vi "PenaltyAttackerRole.vi"(8 "error in (no error)":errorcluster, 9 "Robot in":refnum<class "Robot.lvclass">, 10 "Game in":refnum<class "Game.lvclass">, 11 "PenaltyAttackerRole in":refnum<class "PenaltyAttackerRole.lvclass">) -> (0 "error out":errorcluster, 2 "Robot out":refnum<class "Robot.lvclass">, 3 "PenaltyAttackerRole out":refnum<class "PenaltyAttackerRole.lvclass">)   [LabVIEW 2018, in "PenaltyAttackerRole.lvclass"]
uses:
  PenaltyAttackerRole.lvclass
  C:/Users/Gustavo/Desktop/RoboIMEINTEL/SSL_AI/Role_class/Role.lvclass
  Robot_class/Robot.lvclass
  Game_class/Game.lvclass
  Role_class/Role.lvclass/Role.ctl
  Tacticbook_class/Tacticbook.lvclass/Tacticbook.ctl
  Tacticbook_class/Read PenaltyAttackerTactic.vi
  PenaltyAttackerTactic_class/Read States.vi
  Tacticbook_class/Write PenaltyAttackerTactic.vi
  Role_class/Read Tacticbook.vi
  Role_class/Read tactic_index.vi
  Role_class/Write Tacticbook.vi
  Role_class/Write tactic_index.vi
  Tacticbook_class/Tacticbook.lvclass
  PenaltyAttackerTactic_class/PenaltyAttackerTactic.lvclass
panel:
  out "Game out":refnum<class "Game.lvclass">
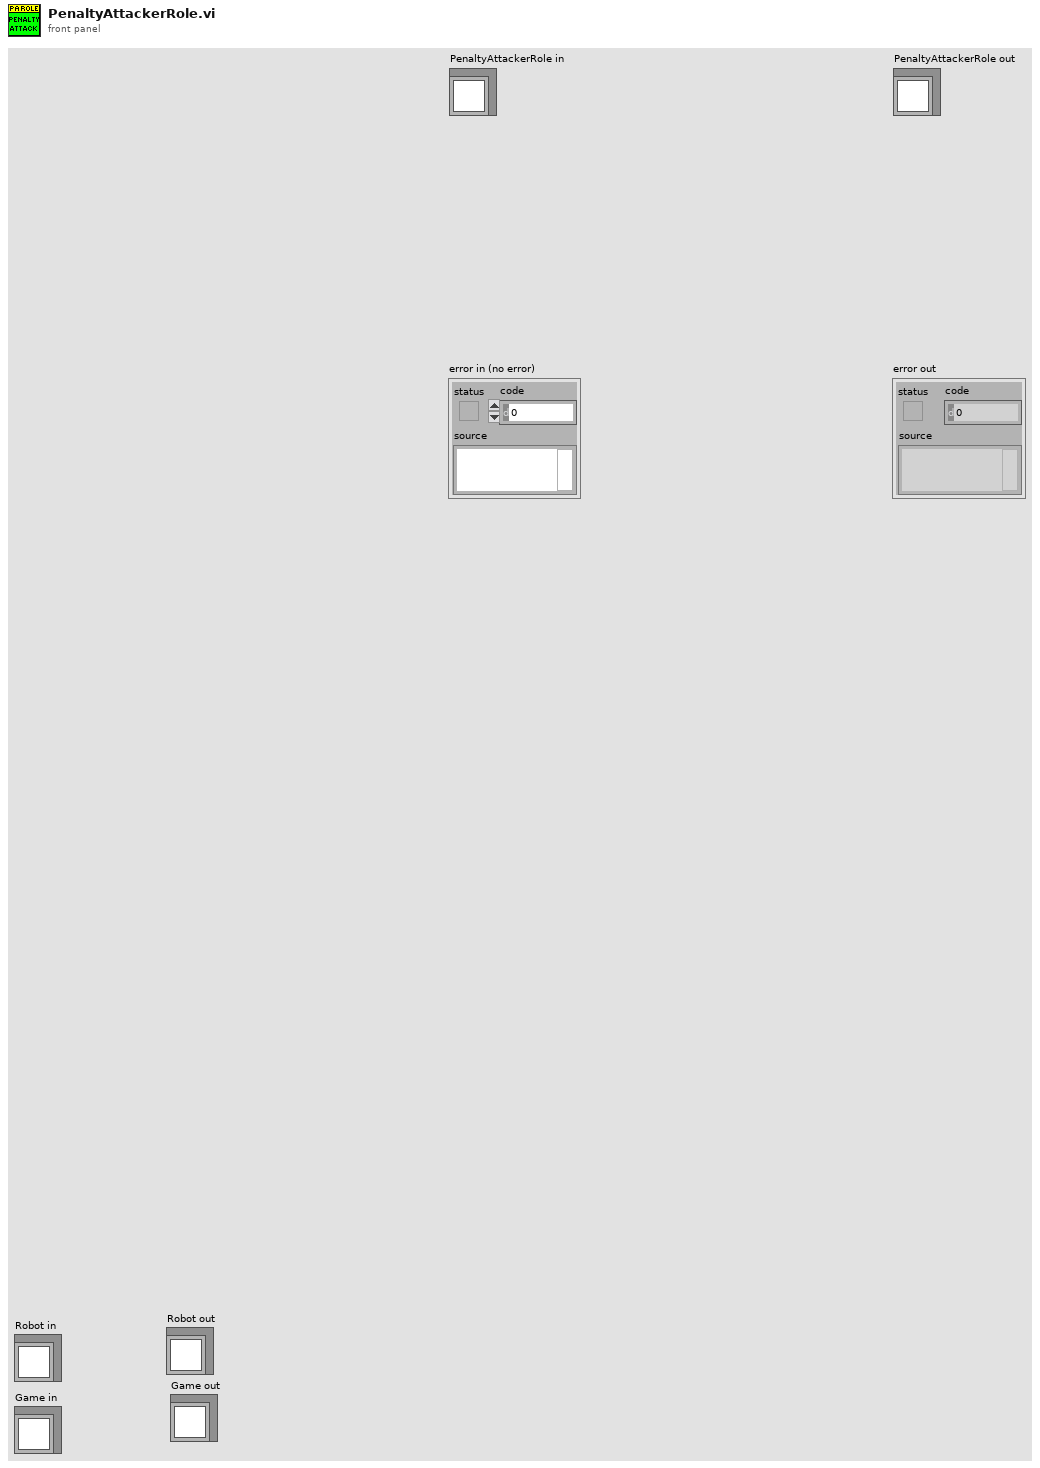
[diagram p1: front panel]
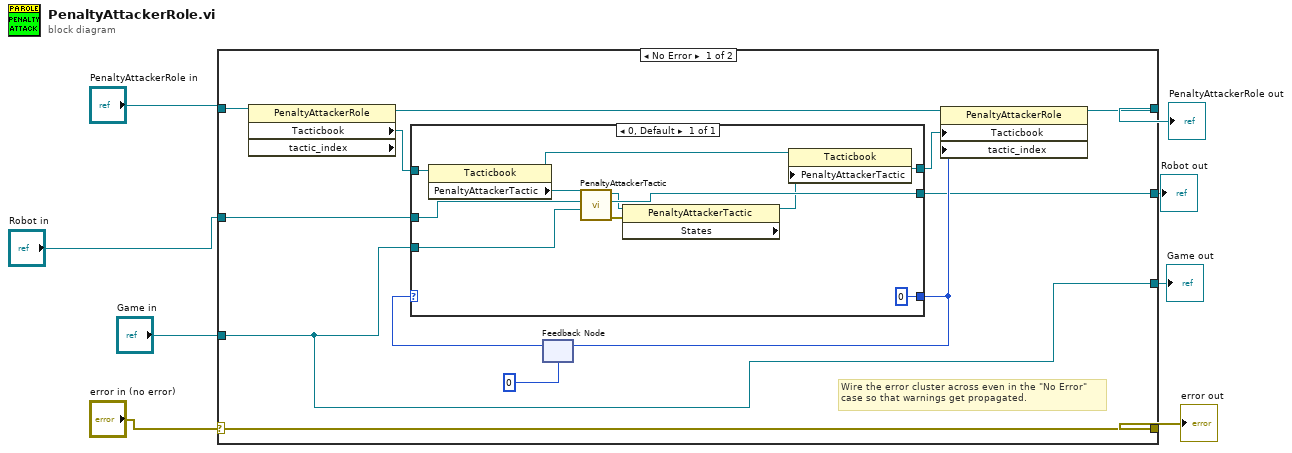
[diagram p0: block diagram]
diagram:
  n1 = case shown="No Error" "error in (no error)" {
    selector: "error in (no error)" -> [w20 w35]
    tunnel: [w20 w35] -> w1
    tunnel: [w18 w34] -> w3
    tunnel: "PenaltyAttackerRole in" -> [w19 w34]
    tunnel: "Robot in" -> [w12 w33]
    tunnel: [w11 w33] -> w8
    tunnel: [w9 w32] -> w7
    tunnel: "Game in" -> [w9 w32]
    frame No Error {
      # "Wire the error cluster across even in the \"No Error\"\ncase so that warnings get propagated."
      n2 = property class="PenaltyAttackerRole" props=["Tacticbook", "tactic_index"](reference=w19) -> (reference out=w17:refnum<class "PenaltyAttackerRole.lvclass">, "Tacticbook"=w14:refnum<class "Tacticbook.lvclass">)  [unwired: 1 in, 2 out]
      n3 = feedback #1(0) -> (w15:i32)
      n4 = case shown="0, Default" w15 {
        tunnel: [0] -> w13
        tunnel: w14 -> [w31]
        tunnel: w12 -> [w24]
        tunnel: [w30] -> w11
        tunnel: [w26] -> w10
        tunnel: w9 -> [w22]
        frame 0, Default {
          n5 = property class="Tacticbook"(reference=w31) -> (reference out=w28:refnum<class "Tacticbook.lvclass">, "PenaltyAttackerTactic"=w25:refnum<class "PenaltyAttackerTactic.lvclass">)  [unwired: 1 in, 1 out]
          n6 = call-dynamic "PenaltyAttackerTactic.vi"("Game"=w22, "Robot"=w24, "PenaltyAttackerTactic in"=w25) -> ("error out"=w29:errorcluster, "Robot out"=w30:refnum<class "Robot.lvclass">, "PenaltyAttackerTactic out"=w23:refnum<class "PenaltyAttackerTactic.lvclass">)  [unwired: 6 in]
          n7 = property class="PenaltyAttackerTactic" props=["States"](reference=w23, error in=w29) -> (reference out=w27:refnum<class "PenaltyAttackerTactic.lvclass">)  [unwired: 2 out]
          n8 = property class="Tacticbook"(reference=w28, "PenaltyAttackerTactic"=w27) -> (reference out=w26:refnum<class "Tacticbook.lvclass">)  [unwired: 1 in, 1 out]
        }
      }
      n9 = feedback-in #1(w13) -> ()
      n10 = property class="PenaltyAttackerRole"(reference=w17, "Tacticbook"=w10, "tactic_index"=w13) -> (reference out=w18:refnum<class "PenaltyAttackerRole.lvclass">)  [unwired: 1 in, 1 out]
    }
    frame Error {
    }
  }
  "error out" <- w1
  "PenaltyAttackerRole out" <- w3
  "Robot out" <- w8
  "Game out" <- w7
